vi "FPGA_task_START.vi"(1 "error in":errorcluster) -> (0 "error out":errorcluster)   [LabVIEW 2015]
uses:
  GLOBAL/Global_FPGA.vi
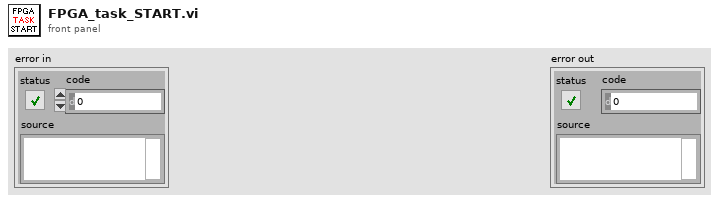
[diagram p1: front panel]
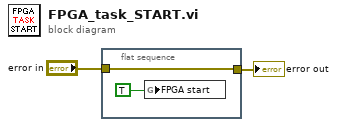
[diagram p0: block diagram]
diagram:
  n1 = flat-sequence {
    tunnel: "error in" -> [w4]
    tunnel: [w4] -> w2
    frame #0 {
      n2 = global write "Global_FPGA.vi" "FPGA start"(TRUE ("Start ANDOR")) -> ()
    }
  }
  "error out" <- w2
